vi "(SubVI)I2C_Ack Check.vi"(8 "에러 입력(에러 없음)":errorcluster, 11 "Read Data":u8[](array[numeric])) -> (0 "에러 출력":errorcluster, 3 "Read Data Out":u8[](array[numeric]))   [LabVIEW 2020]
panel:
  # "(SubVI)I2C_Ack Check.vi By hspark\n\nDescription : 시리얼 통신으로 수신한 I2C 데이터에서 Ack 정보를 확인하여 에러 처리하는 VI\nInput : \n1. Read Data : 시리얼 통신으로 읽은 데이터\n\nOutput : \n1. Read Data Out : Read Data에서 Ack 정보인 앞 2Byte를 제외한 나머지 데이터를 반환\n\nLabVIEW Version : 2020 SP1 이상\n\nNote : 에러 발생 시 에러 코드는 부여하지 않음. 필요 시 사용자 에러 코드 부여할 것.\n\nUpdate : 2021.10.06"
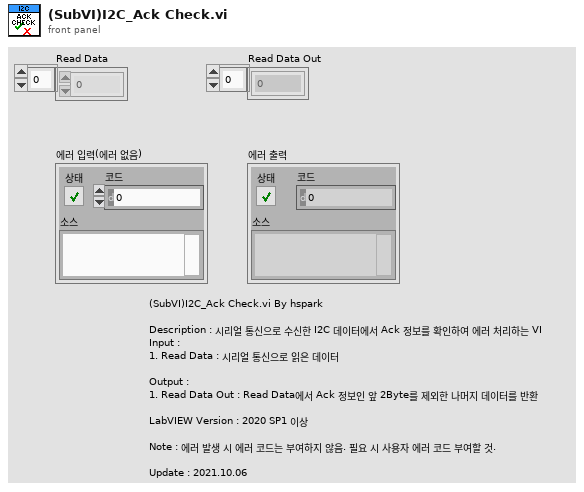
[diagram p1: front panel]
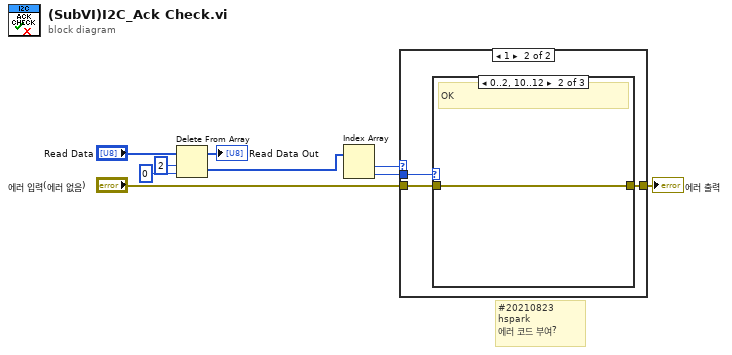
[diagram p0: block diagram]
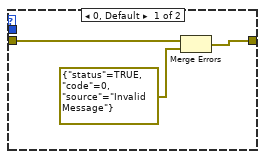
[diagram p2: hidden frame]
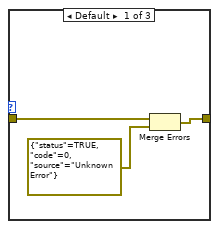
[diagram p3: hidden frame]
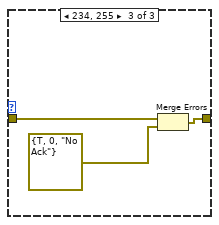
[diagram p4: hidden frame]
diagram:
  # "#20210823\nhspark\n에러 코드 부여?"
  n1 = Delete From Array(array="Read Data", length=2 ("길이"), index=0 ("인덱스")) -> (deleted portion=w2:u8[], array with subset deleted=→"Read Data Out":u8[])
  n2 = Index Array(array=w2) -> (element #1=w7:u8, element #2=w6:u8)  [unwired: 2 in]
  n3 = case shown="1" w7 {
    tunnel: [w11 w15] -> w9
    tunnel: "에러 입력(에러 없음)" -> [w12 w14]
    tunnel: w6 -> [_ w13]
    frame 0, Default {
      n4 = Merge Errors(w12, errorcluster {"status"=TRUE, "code"=0, "source"="Invalid Message"} ("error IO")) -> (w11:errorcluster)
    }
    frame 1 {
      n5 = case shown="0..2, 10..12" w13 {
        tunnel: w14 -> [w18 w19 w22]
        tunnel: [w17 w19 w21] -> w15
        frame Default {
          n6 = Merge Errors(w18, errorcluster {"status"=TRUE, "code"=0, "source"="Unknown Error"} ("에러 입력")) -> (w17:errorcluster)
        }
        frame 0..2, 16..18 {
          # "OK"
        }
        frame 234, 255 {
          n7 = Merge Errors(w22, errorcluster {"status"=TRUE, "code"=0, "source"="No Ack"} ("에러 입력")) -> (w21:errorcluster)
        }
      }
    }
  }
  "에러 출력" <- w9
